vi "Configure Clock Recovery Method.vi"(0 "VISA resource name":refnum<visa-resource-name>, 1 "Clock":T1={"Clock Edge (0: Rising)"=0, "Clock Multiplier (1)"=1, "Clock Frequency (2.5E+9 Hz)"=2500000000.0} {"Clock Edge (0: Rising)" items=["Rising", "Falling", "Both"]}, 2 "Track Frequency (2.5E+9 Hz)":dbl=2500000000.0, 3 "Baud Rate (1E+7 bits/s)":dbl=10000000.0 format="%#.3g", 5 "Measurement Source (1: Channel 1)":i32(ring)=1 items=["Channel 1"=1, "Channel 2"=2, "Channel 3"=3, "Channel 4"=4, "Function 1"=5, "Function 2"=6, "Function 3"=7, "Function 4"=8, "Memory 1"=9, "Memory 2"=10, "Memory 3"=11, "Memory 4"=12], 7 "Clock Recovery Method (4: Constant Frequency)":i32(ring)=4 items=["PCI Express", "Fibre Channel", "First Order PLL", "Second Order PLL", "Constant Frequency", "Explicit Clock", "Explicit First Order PLL", "Explicit Second Order PLL", "FlexRay Receiver", "FlexRay Transmitter", "Equalized First Order PLL", "Equalized Second Order PLL"], 9 "Data Rate and Bandwidth":T2={"Nominal Data Rate (2.5E+9 Hz)"=2500000000.0, "Loop Bandwidth (1.4997E+6 Hz)"=1499700.0, "Data Rate Type (0: Fully Automatic)"=0, "Data Bits (0: Both)"=0} {"Data Bits (0: Both)" items=["Both", "Deemphasis", "Transition"]; "Data Rate Type (0: Fully Automatic)" items=["Fully Automatic", "Semi-Automatic", "Manual"]}, 11 "error in (no error)":errorcluster, 12 "Fibre Channel (0: FC1063)":i32(ring) items=["FC1063", "FC2125", "FC425"], 13 "Damping Factor (1 bits/s)":dbl=1.0 format="%#.3g") -> (4 "VISA resource name out":refnum<visa-resource-name>, 15 "error out":errorcluster)   [LabVIEW 2020, in "Agilent 90000 Series.lvlib"]
doc: "Configures the clock recovery method parameters."
uses:
  Agilent 90000 Series.lvlib
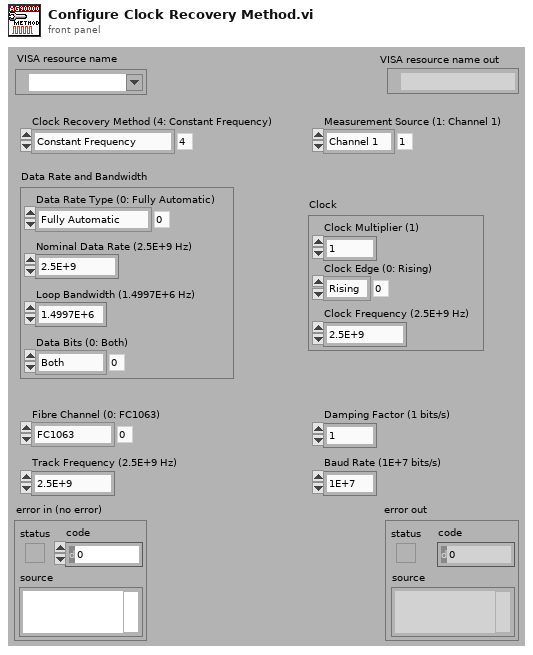
[diagram p1: front panel]
types:
  T1 = cluster{"Clock Edge (0: Rising)":i32, "Clock Multiplier (1)":i32, "Clock Frequency (2.5E+9 Hz)":dbl}
  T2 = cluster{"Nominal Data Rate (2.5E+9 Hz)":dbl, "Loop Bandwidth (1.4997E+6 Hz)":dbl, "Data Rate Type (0: Fully Automatic)":i32, "Data Bits (0: Both)":i32}
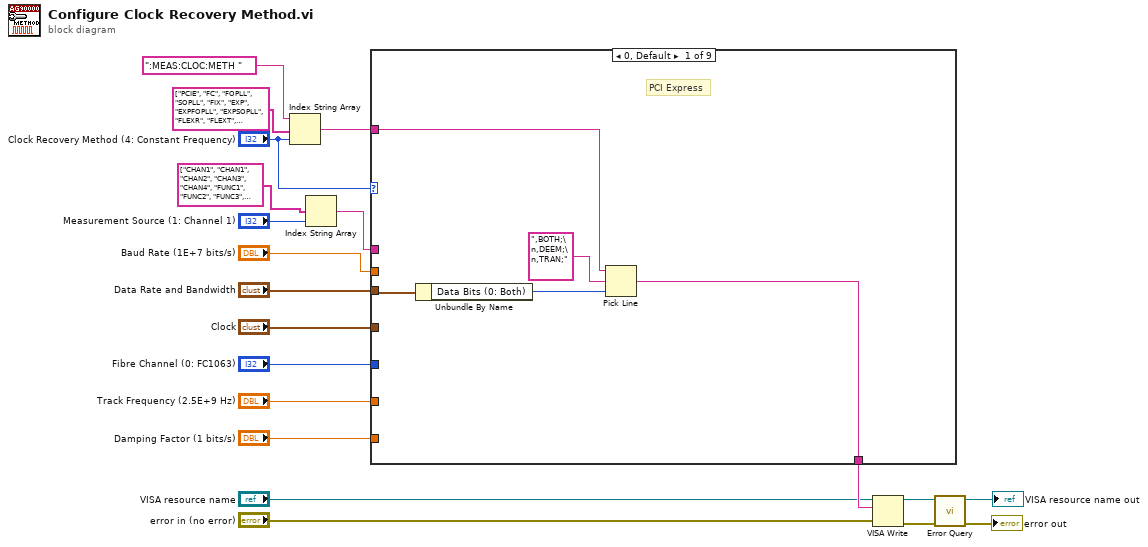
[diagram p0: block diagram]
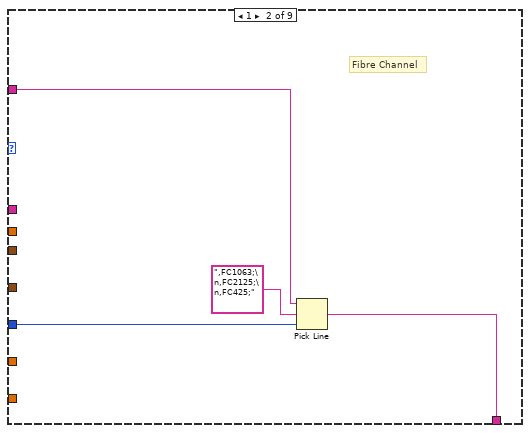
[diagram p2: hidden frame]
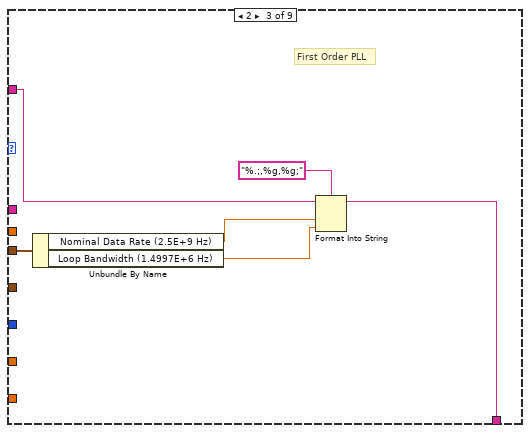
[diagram p3: hidden frame]
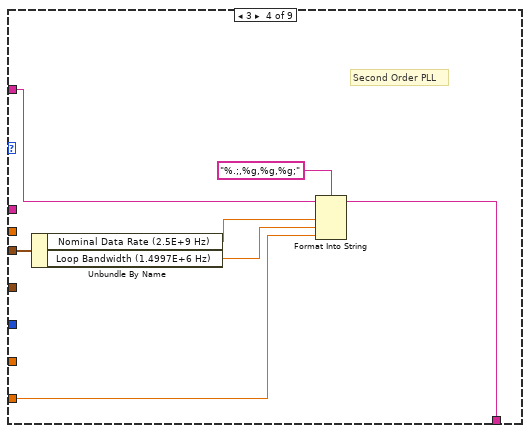
[diagram p4: hidden frame]
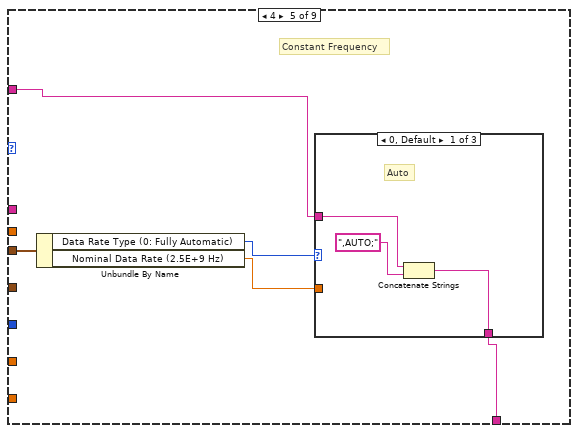
[diagram p5: hidden frame]
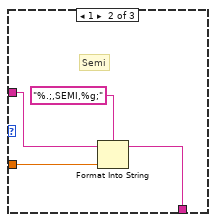
[diagram p6: hidden frame]
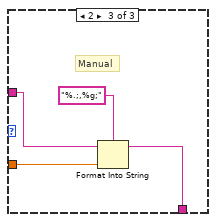
[diagram p7: hidden frame]
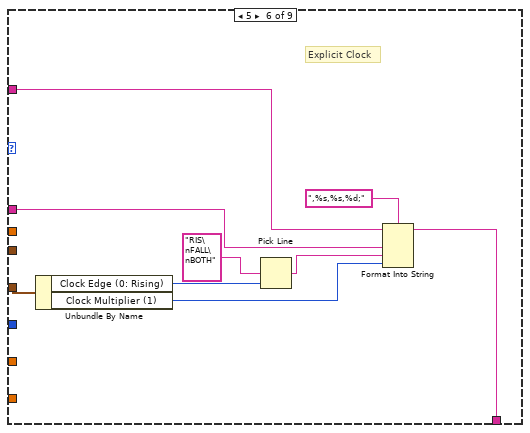
[diagram p8: hidden frame]
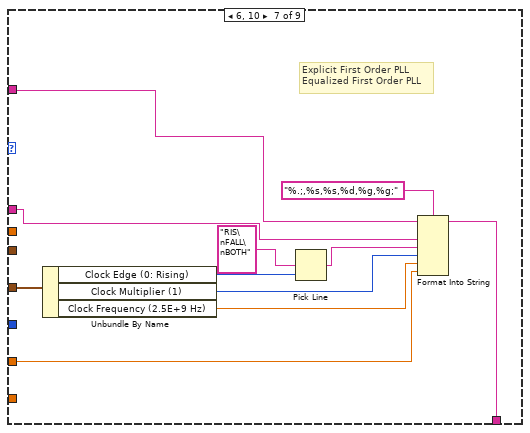
[diagram p9: hidden frame]
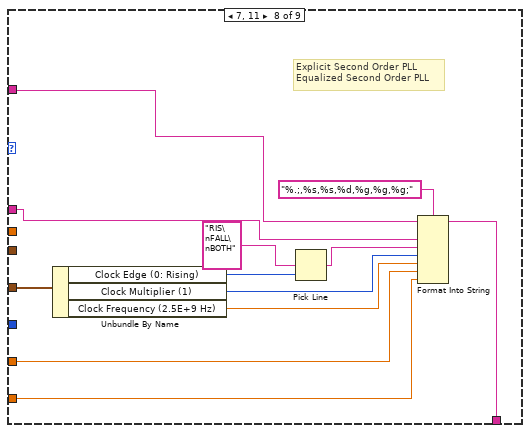
[diagram p10: hidden frame]
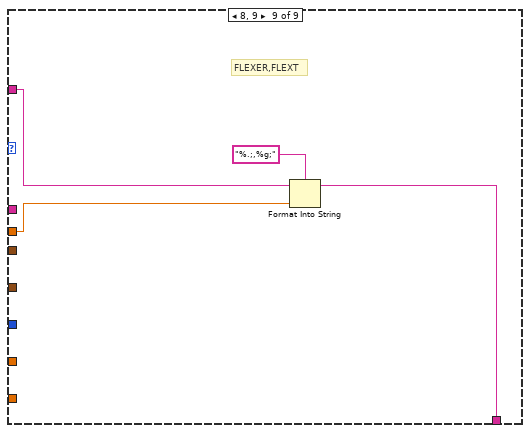
[diagram p11: hidden frame]
diagram:
  n1 = Index String Array(1:"Clock Recovery Method (4: Constant Frequency)", 2:string[] ["PCIE", "FC", "FOPLL", "SOPLL", "FIX", "EXP", "EXPFOPLL", "EXPSOPLL", "FLEXR", "FLEXT", "EQFOPLL", "EQSOPLL"], 3:":MEAS:CLOC:METH ") -> (0:w14:string)
  n2 = Index String Array(1:"Measurement Source (1: Channel 1)", 2:string[] ["CHAN1", "CHAN1", "CHAN2", "CHAN3", "CHAN4", "FUNC1", "FUNC2", "FUNC3", "FUNC4", "WMEM1", "WMEM2", "WMEM3", "WMEM4"] ("subarray 2")) -> (0:w7:string)  [unwired: 1 out]
  n3 = case shown="0, Default" "Clock Recovery Method (4: Constant Frequency)" {
    tunnel: w14 -> [w22 w27 w34 w41 w45 w60 w71 w83 w93]
    tunnel: "Data Rate and Bandwidth" -> [w25 _ w35 w42 w47 _ _ _ _]
    tunnel: [w21 w26 w30 w37 w44 w61 w68 w80 w91] -> w11
    tunnel: "Fibre Channel (0: FC1063)" -> [_ w28 _ _ _ _ _ _ _]
    tunnel: "Damping Factor (1 bits/s)" -> [_ _ _ w36 _ _ _ w79 _]
    tunnel: w7 -> [_ _ _ _ _ w59 w73 w85 _]
    tunnel: "Clock" -> [_ _ _ _ _ w67 w74 w86 _]
    tunnel: "Baud Rate (1E+7 bits/s)" -> [_ _ _ _ _ _ _ _ w92]
    tunnel: "Track Frequency (2.5E+9 Hz)" -> [_ _ _ _ _ _ w70 w82 _]
    frame 0, Default {
      # "PCI Express"
      n4 = Unbundle By Name(w25) -> ("Data Bits (0: Both)"=w24:i32)
      n5 = Pick Line(string ("")=w22, multi-line string=",BOTH;\n,DEEM;\n,TRAN;", line index=w24) -> (output string=w21:string)
    }
    frame 1 {
      # "Fibre Channel"
      n6 = Pick Line(string ("")=w27, multi-line string=",FC1063;\n,FC2125;\n,FC425;", line index=w28) -> (output string=w26:string)
    }
    frame 2 {
      # "First Order PLL"
      n7 = Unbundle By Name(w35) -> ("Nominal Data Rate (2.5E+9 Hz)"=w32:dbl, "Loop Bandwidth (1.4997E+6 Hz)"=w31:dbl)
      n8 = Format Into String(format string="%.;,%g,%g;", initial string=w34, w32, w31) -> (resulting string=w30:string)  [unwired: 1 in, 1 out]
    }
    frame 3 {
      # "Second Order PLL"
      n9 = Unbundle By Name(w42) -> ("Nominal Data Rate (2.5E+9 Hz)"=w39:dbl, "Loop Bandwidth (1.4997E+6 Hz)"=w38:dbl)
      n10 = Format Into String(format string="%.;,%g,%g,%g;", initial string=w41, w39, w38, w36) -> (resulting string=w37:string)  [unwired: 1 in, 1 out]
    }
    frame 4 {
      # "Constant Frequency"
      n11 = Unbundle By Name(w47) -> ("Data Rate Type (0: Fully Automatic)"=w46:i32, "Nominal Data Rate (2.5E+9 Hz)"=w43:dbl)
      n12 = case shown="0, Default" w46 {
        tunnel: w45 -> [w49 w53 w57]
        tunnel: [w50 w52 w56] -> w44
        tunnel: w43 -> [_ w51 w55]
        frame 0, Default {
          # "Auto"
          n13 = Concatenate Strings(w49, ",AUTO;" ("format string")) -> (w50:string)
        }
        frame 1 {
          # "Semi"
          n14 = Format Into String(format string="%.;,SEMI,%g;", initial string=w53, w51) -> (resulting string=w52:string)  [unwired: 1 in, 1 out]
        }
        frame 2 {
          # "Manual"
          n15 = Format Into String(format string="%.;,%g;", initial string=w57, w55) -> (resulting string=w56:string)  [unwired: 1 in, 1 out]
        }
      }
    }
    frame 5 {
      # "Explicit Clock"
      n16 = Unbundle By Name(w67) -> ("Clock Edge (0: Rising)"=w66:i32, "Clock Multiplier (1)"=w63:i32)
      n17 = Pick Line(multi-line string="RIS\nFALL\nBOTH", line index=w66) -> (output string=w62:string)  [unwired: 1 out]
      n18 = Format Into String(format string=",%s,%s,%d;", initial string=w60, w59, w62, w63) -> (resulting string=w61:string)  [unwired: 1 in, 1 out]
    }
    frame 6, 10 {
      # "Explicit First Order PLL\nEqualized First Order PLL"
      n19 = Unbundle By Name(w74) -> ("Clock Edge (0: Rising)"=w78:i32, "Clock Multiplier (1)"=w76:i32, "Clock Frequency (2.5E+9 Hz)"=w69:dbl)
      n20 = Pick Line(multi-line string="RIS\nFALL\nBOTH", line index=w78) -> (output string=w75:string)  [unwired: 1 out]
      n21 = Format Into String(format string="%.;,%s,%s,%d,%g,%g;", initial string=w71, w73, w75, w76, w69, w70) -> (resulting string=w68:string)  [unwired: 1 in, 1 out]
    }
    frame 7, 11 {
      # "Explicit Second Order PLL\nEqualized Second Order PLL"
      n22 = Unbundle By Name(w86) -> ("Clock Edge (0: Rising)"=w90:i32, "Clock Multiplier (1)"=w88:i32, "Clock Frequency (2.5E+9 Hz)"=w81:dbl)
      n23 = Pick Line(multi-line string="RIS\nFALL\nBOTH", line index=w90) -> (output string=w87:string)  [unwired: 1 out]
      n24 = Format Into String(format string="%.;,%s,%s,%d,%g,%g,%g;", initial string=w83, w85, w87, w88, w81, w82, w79) -> (resulting string=w80:string)  [unwired: 1 in, 1 out]
    }
    frame 8, 9 {
      # "FLEXER,FLEXT"
      n25 = Format Into String(format string="%.;,%g;", initial string=w93, w92) -> (resulting string=w91:string)  [unwired: 1 in, 1 out]
    }
  }
  n26 = VISA Write(VISA resource name="VISA resource name", write buffer=w11, error in (no error)="error in (no error)") -> (VISA resource name out=w18:refnum<visa-resource-name>, error out=w17:errorcluster)  [unwired: 1 out]
  n27 = call "Error Query.vi"("error in (no error)"=w17, "VISA resource name"=w18) -> ("error out"=→"error out":errorcluster, "VISA resource name out"=→"VISA resource name out":refnum<visa-resource-name>)  [unwired: 8 out]
